vi "stage_control.vi"(8 "error in (no error)":errorcluster, 9 "Close Stage":bool=TRUE, 10 "Initialize Stage":bool=TRUE, 11 "VISA in":refnum<visa-resource-name>="COM5") -> (0 "error out":errorcluster, 3 "VISA out":refnum<visa-resource-name>)   [LabVIEW 2018]
panel:
  out "Numeric status":dbl
  in  "Flip Mirror":sgl(ring) items=["EMCCD Camera"=0, "Wavefront sensor"=5]
  in  "flip mirror button":bool
  in  "stop":bool
  in  "baud rate (9600)":u32=9600
  in  "Z step (10=1um)":dbl=1.0
  in  "up":bool
  in  "down":bool
  in  "XY step (10=1um)":dbl=1.0
  in  "back":bool
  in  "front":bool
  in  "left":bool
  in  "right":bool
  # "Add function: get current  XYZ position"
  # "Sample Stage"
  # "WF switch"
  # "Defocus: +"
  # "Old Control (disabled)"
  # "Tilt 1/X: +"
  # "Click to switch mirror position"
  # "Tilt 2/Y: -"
  # "EMCCD: 0"
  # "Wavefront Sensor: 5"
  # "WFS no tilt: X502, Y520 @EMCCD"
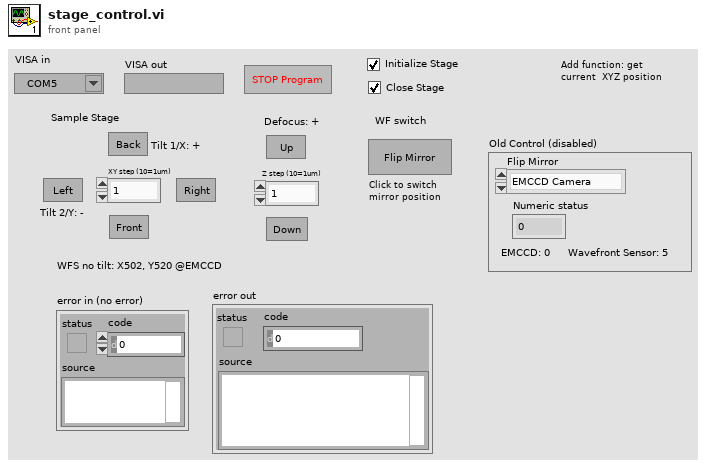
[diagram p1: front panel]
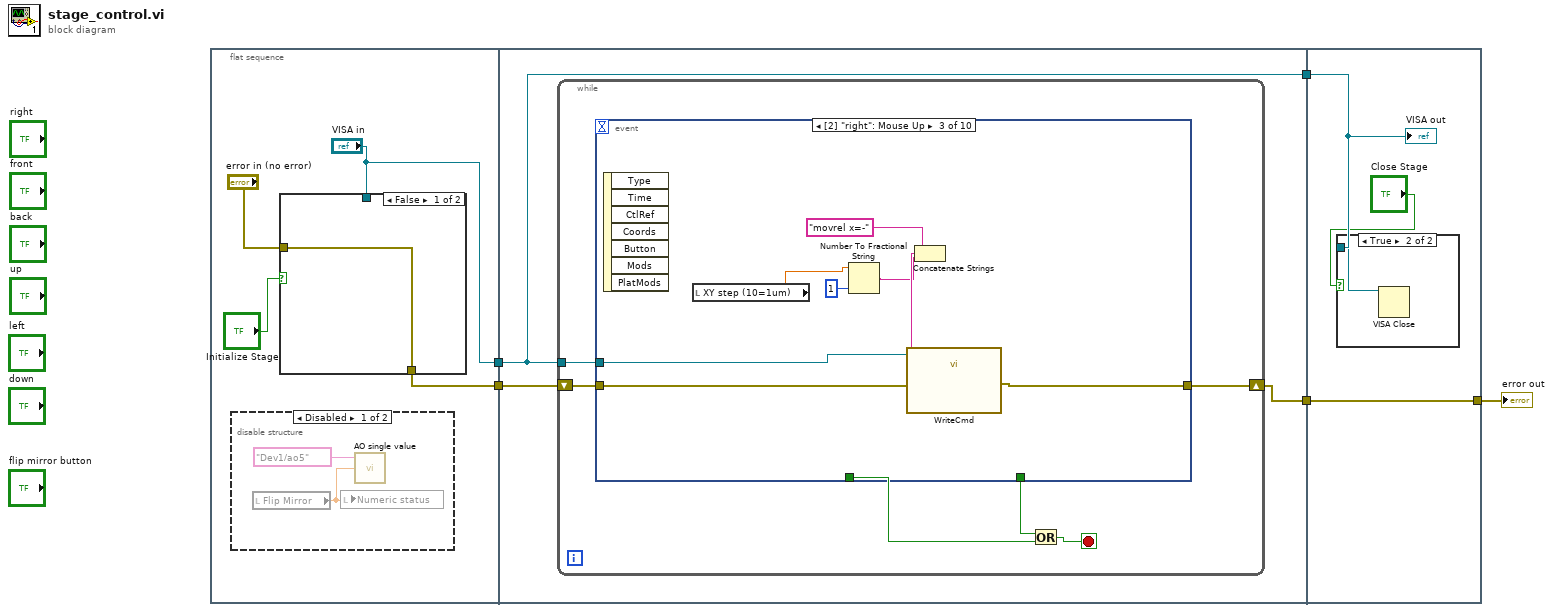
[diagram p0: block diagram]
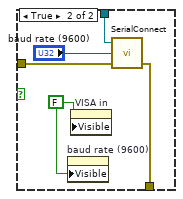
[diagram p2: hidden frame]
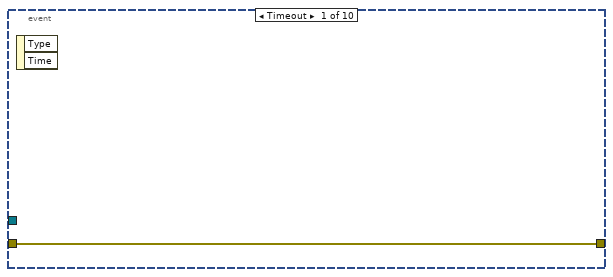
[diagram p4: hidden frame]
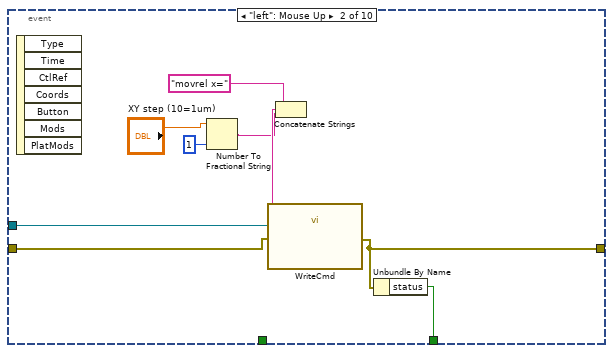
[diagram p5: hidden frame]
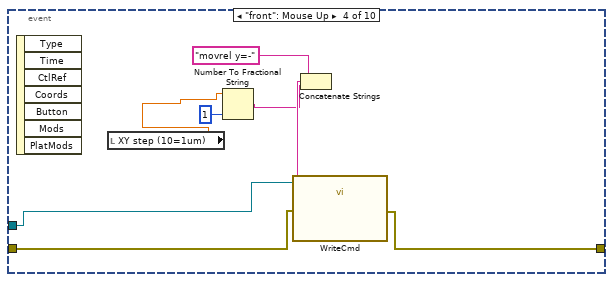
[diagram p6: hidden frame]
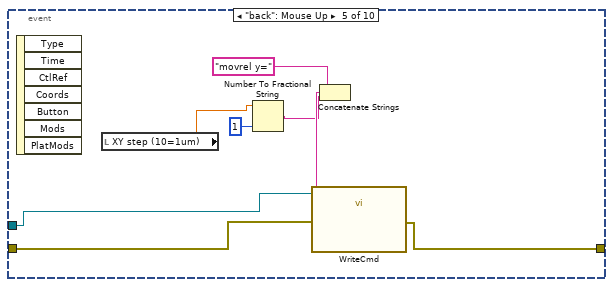
[diagram p7: hidden frame]
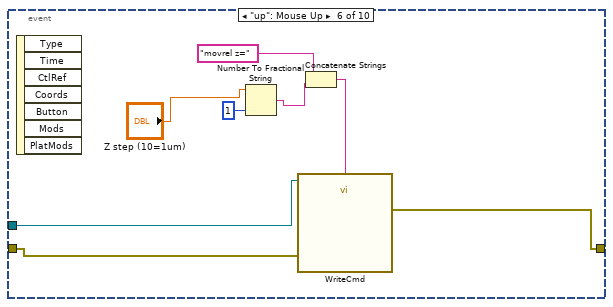
[diagram p8: hidden frame]
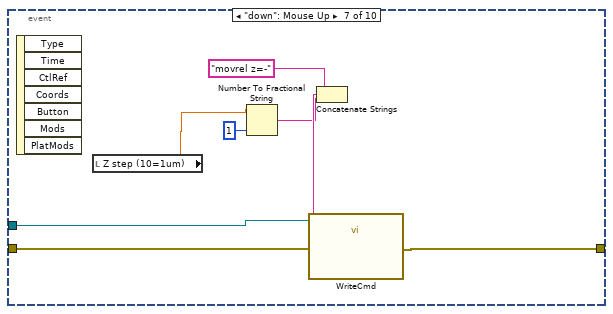
[diagram p9: hidden frame]
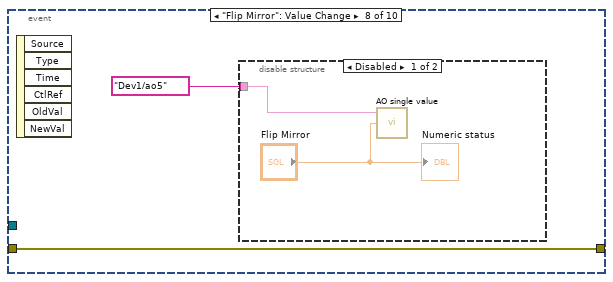
[diagram p10: hidden frame]
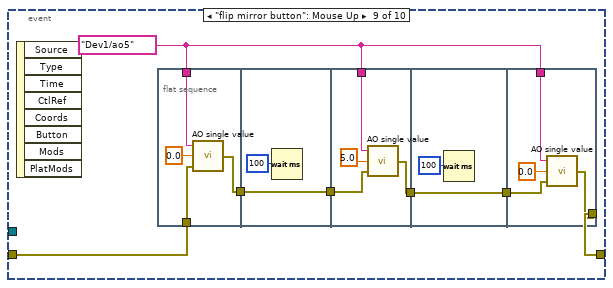
[diagram p12: hidden frame]
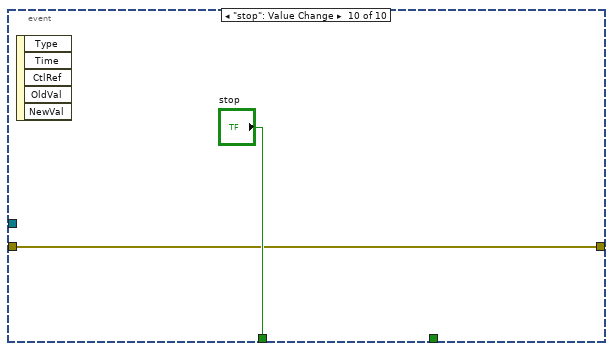
[diagram p13: hidden frame]
diagram:
  n1 = flat-sequence {
    tunnel: [w8] -> w5
    tunnel: ["VISA in"] -> w2
    tunnel: w5 -> [w20]
    tunnel: [w19] -> w3
    tunnel: w2 -> [w18]
    tunnel: [w18] -> w1
    tunnel: [w108] -> w4
    tunnel: w3 -> [w108]
    tunnel: w1 -> [w107]
    frame #0 {
      n2 = disable-structure shown="Disabled" {
        frame Disabled {
          n3 = local read "Flip Mirror"() -> (w16:sgl)
          n4 = local write "Numeric status"(w16) -> ()
          n5 = call "AO single value.vi"("data"=w16, "physical channels"=tag "Dev1/ao5") -> ()  [unwired: 1 in, 1 out]
        }
        frame Enabled {
        }
      }
      n6 = case shown="False" "Initialize Stage" {
        tunnel: "error in (no error)" -> [w10 w13]
        tunnel: [w10 w12] -> w8
        tunnel: "VISA in" -> [_ w11]
        frame False {
        }
        frame True {
          w14 = FALSE ("Visible")
          n7 = property on="baud rate (9600)" class="DigNum (strict)"("Visible"=w14) -> ()  [unwired: 2 in, 2 out]
          n8 = property on="VISA in" class="VISAName"("Visible"=w14) -> ()  [unwired: 2 in, 2 out]
          n9 = call "SerialConnect.vi"("error in (no error)"=w13, "baud rate (9600)"="baud rate (9600)", "VISA resource name"=w11) -> ("error out"=w12:errorcluster)  [unwired: 2 out]
        }
      }
    }
    frame #1 {
      n10 = while {
        shift-right: [w22] -> w19
        shift-left: w20 -> [w23]
        tunnel: w18 -> [w21]
        stop <- w26 stop-if-true
        n11 = event shown="[2] \"right\": Mouse Up" {
          selector: _ -> [_ _ _ _ _ _ _ _ _ _]
          dyn-events: _ -> [_ _ _ _ _ _ _ _ _ _]
          timeout: _ -> [_ _ _ _ _ _ _ _ _ _]
          tunnel: [_ _ _ _ _ _ _ _ _ "stop"] -> w25
          tunnel: [_ w34 _ _ _ _ _ _ _ _] -> w24
          tunnel: w23 -> [w27 w33 w42 w50 w58 w66 w74 w77 w82 w104]
          tunnel: [w27 w32 w41 w49 w57 w65 w73 w77 w81 w104] -> w22
          tunnel: w21 -> [_ w31 w40 w48 w56 w64 w72 _ _ _]
          event Timeout {
            n12 = event-data() -> ()  [unwired: 1 in, 2 out]
          }
          event "left": Mouse Up {
            n13 = event-data() -> ()  [unwired: 1 in, 7 out]
            n14 = Number To Fractional String(number="XY step (10=1um)", precision (6)=1) -> (F-format string=w29:string)  [unwired: 2 in]
            n15 = Concatenate Strings("movrel x=", w29) -> (w35:string)
            n16 = call "WriteCmd.vi"("error IO"=w33, "Command"=w35, "VISA resource name"=w31) -> ("error"=w32:errorcluster)  [unwired: 1 out]
            n17 = Unbundle By Name(w32) -> ("status"=w34:bool)
          }
          event "right": Mouse Up {
            n18 = event-data() -> ()  [unwired: 1 in, 7 out]
            n19 = local read "XY step (10=1um)"() -> (w37:dbl)
            n20 = Number To Fractional String(number=w37, precision (6)=1) -> (F-format string=w38:string)  [unwired: 2 in]
            n21 = Concatenate Strings("movrel x=-", w38) -> (w43:string)
            n22 = call "WriteCmd.vi"("error IO"=w42, "Command"=w43, "VISA resource name"=w40) -> ("error"=w41:errorcluster)  [unwired: 1 out]
          }
          event "front": Mouse Up {
            n23 = event-data() -> ()  [unwired: 1 in, 7 out]
            n24 = local read "XY step (10=1um)"() -> (w45:dbl)
            n25 = Number To Fractional String(number=w45, precision (6)=1) -> (F-format string=w46:string)  [unwired: 2 in]
            n26 = Concatenate Strings("movrel y=-", w46) -> (w51:string)
            n27 = call "WriteCmd.vi"("error IO"=w50, "Command"=w51, "VISA resource name"=w48) -> ("error"=w49:errorcluster)  [unwired: 1 out]
          }
          event "back": Mouse Up {
            n28 = event-data() -> ()  [unwired: 1 in, 7 out]
            n29 = local read "XY step (10=1um)"() -> (w53:dbl)
            n30 = Number To Fractional String(number=w53, precision (6)=1) -> (F-format string=w54:string)  [unwired: 2 in]
            n31 = Concatenate Strings("movrel y=", w54) -> (w59:string)
            n32 = call "WriteCmd.vi"("error IO"=w58, "Command"=w59, "VISA resource name"=w56) -> ("error"=w57:errorcluster)  [unwired: 1 out]
          }
          event "up": Mouse Up {
            n33 = event-data() -> ()  [unwired: 1 in, 7 out]
            n34 = Number To Fractional String(number="Z step (10=1um)", precision (6)=1) -> (F-format string=w62:string)  [unwired: 2 in]
            n35 = Concatenate Strings("movrel z=", w62) -> (w67:string)
            n36 = call "WriteCmd.vi"("error IO"=w66, "Command"=w67, "VISA resource name"=w64) -> ("error"=w65:errorcluster)  [unwired: 1 out]
          }
          event "down": Mouse Up {
            n37 = event-data() -> ()  [unwired: 1 in, 7 out]
            n38 = local read "Z step (10=1um)"() -> (w69:dbl)
            n39 = Number To Fractional String(number=w69, precision (6)=1) -> (F-format string=w70:string)  [unwired: 2 in]
            n40 = Concatenate Strings("movrel z=-", w70) -> (w75:string)
            n41 = call "WriteCmd.vi"("error IO"=w74, "Command"=w75, "VISA resource name"=w72) -> ("error"=w73:errorcluster)  [unwired: 1 out]
          }
          event "Flip Mirror": Value Change {
            n42 = event-data() -> ()  [unwired: 1 in, 6 out]
            n43 = disable-structure shown="Disabled" {
              disable-tunnel: tag "Dev1/ao5" ("physical channels") -> [w79 _]
              frame Disabled {
                n44 = call "AO single value.vi"("data"="Flip Mirror", "physical channels"=w79) -> ()  [unwired: 1 in, 1 out]
                "Numeric status" <- "Flip Mirror"
              }
              frame Enabled {
              }
            }
          }
          event "flip mirror button": Mouse Up {
            w83 = tag "Dev1/ao5" ("physical channels")
            n45 = event-data() -> ()  [unwired: 1 in, 8 out]
            n46 = flat-sequence {
              tunnel: [w91] -> w86
              tunnel: w83 -> [w89]
              tunnel: w82 -> [w88]
              tunnel: [w92] -> w87
              tunnel: w86 -> [w92]
              tunnel: w87 -> [w96]
              tunnel: [w95] -> w84
              tunnel: w83 -> [w94]
              tunnel: [w98] -> w85
              tunnel: w84 -> [w98]
              tunnel: w85 -> [w102]
              tunnel: w83 -> [w101]
              tunnel: [w100] -> w81
              frame #0 {
                n47 = call "AO single value.vi"("error in"=w88, "data"=0.0, "physical channels"=w89) -> ("error out"=w91:errorcluster)
              }
              frame #1 {
                n48 = Wait (ms)(milliseconds to wait=u32 100) -> ()  [unwired: 1 out]
              }
              frame #2 {
                n49 = call "AO single value.vi"("error in"=w96, "data"=5.0, "physical channels"=w94) -> ("error out"=w95:errorcluster)
              }
              frame #3 {
                n50 = Wait (ms)(milliseconds to wait=u32 100) -> ()  [unwired: 1 out]
              }
              frame #4 {
                n51 = call "AO single value.vi"("error in"=w102, "data"=0.0, "physical channels"=w101) -> ("error out"=w100:errorcluster)
              }
            }
          }
          event "stop": Value Change {
            n52 = event-data() -> ()  [unwired: 1 in, 5 out]
          }
        }
        n53 = Or(x=w24, y=w25) -> (x .or. y?=w26:bool)
      }
    }
    frame #2 {
      n54 = case shown="True" "Close Stage" {
        tunnel: w107 -> [_ w109]
        frame False {
        }
        frame True {
          n55 = VISA Close(VISA resource name=w109) -> ()  [unwired: 1 in, 1 out]
        }
      }
      "VISA out" <- w107
    }
  }
  "error out" <- w4
